vi "getAllChannels.vi"(8 "error in (no error)":errorcluster, 11 "ChannelArray.lvclass in":refnum<class "ChannelArray.lvclass">) -> (0 "error out":errorcluster, 2 "channels":refnum<class "Channel.lvclass">[](array[class]), 3 "ChannelArray.lvclass out":refnum<class "ChannelArray.lvclass">)   [LabVIEW 2009, in "Tools.lvlib" / "DatabaseHelpers.lvlib" / "ChannelArray.lvclass"]
uses:
  ChannelArray.lvclass
  Channel/Channel.lvclass
  ChannelArray.lvclass/ChannelArray.ctl
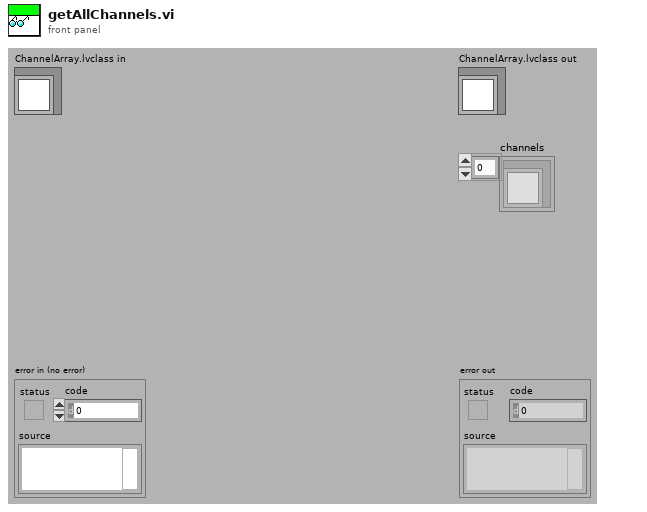
[diagram p1: front panel]
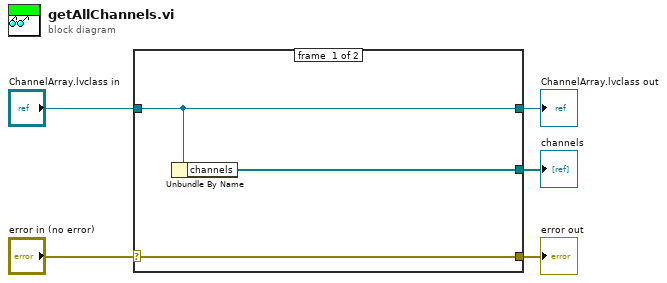
[diagram p0: block diagram]
diagram:
  n1 = case shown="No Error" "error in (no error)" {
    selector: "error in (no error)" -> [w8 w9]
    tunnel: [w8 w9] -> w4
    tunnel: [w7 w10] -> w2
    tunnel: "ChannelArray.lvclass in" -> [w7 w10]
    tunnel: [w6 _] -> w1
    frame #0 {
      n2 = Unbundle By Name(w7) -> ("channels"=w6:refnum<class "Channel.lvclass">[])
    }
    frame #1 {
    }
  }
  "error out" <- w4
  "ChannelArray.lvclass out" <- w2
  "channels" <- w1
